vi "relay board with 8 bit word.vi"() -> ()   [LabVIEW 2013]
panel:
  in  "Array":u8[](array[slide]) scale=0.0..255.0
  out "Waveform Chart":dynamicdata(graph) caption="Voltage"
  out "Output":dbl
  out "Input":dbl
  in  "Slide":dbl(slide) scale=-10.0..10.0
  in  "stop":bool
  # "65"
  # "66"
  # "67"
  # "68"
  # "69"
  # "70"
  # "71"
  # "72"
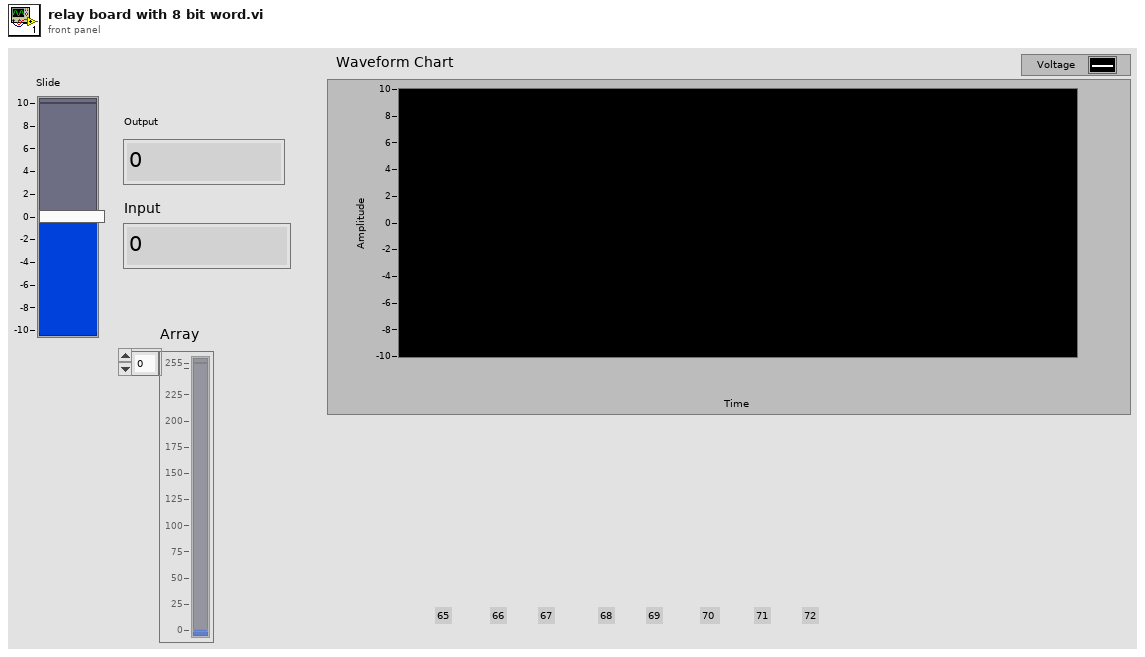
[diagram p1: front panel]
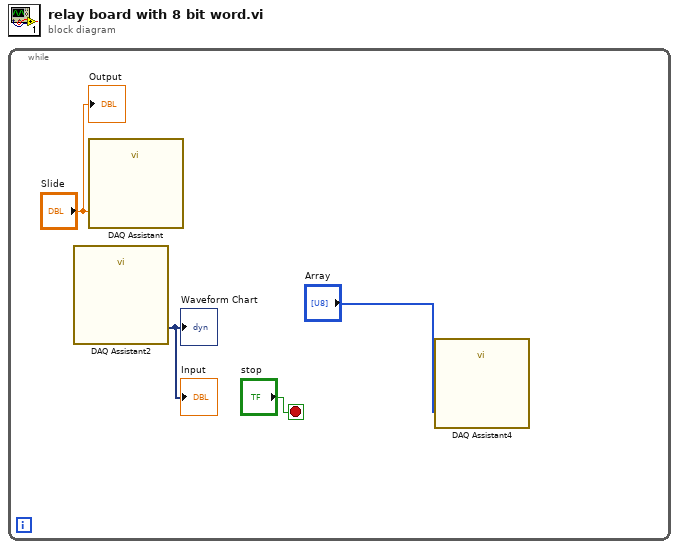
[diagram p0: block diagram]
diagram:
  n1 = while {
    stop <- "stop" stop-if-true
    n2 = call "DAQ Assistant2"() -> ("data"=→"Input" →"Waveform Chart":dynamicdata)  [unwired: 16 in, 3 out]
    n3 = call "DAQ Assistant"("data"="Slide") -> ()  [unwired: 17 in, 2 out]
    n4 = call "DAQ Assistant4"("data"="Array") -> ()  [unwired: 17 in, 2 out]
    "Output" <- "Slide"
  }
